vi "Coord window-Move to XY.vi"(8 "error in (no error)":errorcluster) -> (0 "error out":errorcluster)   [LabVIEW 2013]
uses:
  Globals/Coord window-Globals.vi
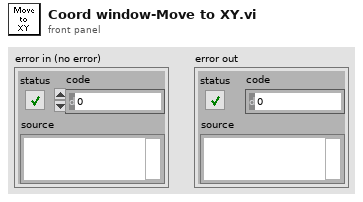
[diagram p1: front panel]
types:
  T1 = typedef "Coordinate list window refs.ctl" = cluster{"Window Name (i.e. Key)":string, "menu reference":refnum<k9>, "VI's reference":refnum<vi>, "Pane 1":refnum<vi>, "Pane 2":refnum<vi>, "Coord Listbox":refnum<vi>, "File name":refnum<vi>, "Picture Map":refnum<vi>, "Stage XYZ Position ind.":refnum<vi>}
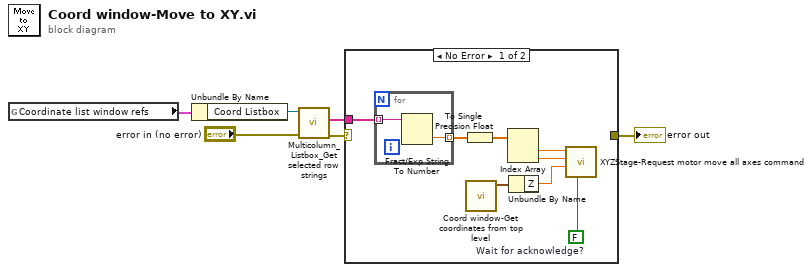
[diagram p0: block diagram]
diagram:
  n1 = global read "Coord window-Globals.vi" "Coordinate list window refs"() -> (w5:T1)
  n2 = Unbundle By Name(w5) -> ("Coord Listbox"=w4:refnum<vi>)
  n3 = call "Multicolumn_Listbox_Get selected row strings.vi"("error in (no error)"="error in (no error)", "MulticolumnListbox in"=w4) -> ("error out"=w3:errorcluster, "Selected row strings"=w6:string[])  [unwired: 7 in, 1 out]
  n4 = case shown="No Error" w3 {
    selector: w3 -> [_ w17]
    tunnel: w6 -> [w8 _]
    tunnel: [_ w17] -> w2
    frame No Error {
      w14 = FALSE  # Wait for acknowledge?
      n5 = for {
        tunnel: w8 -> [w16] mode=indexing
        tunnel: [w15] -> w9 mode=indexing
        n6 = Fract/Exp String To Number(string=w16) -> (number=w15:dbl)  [unwired: 3 in, 1 out]
      }
      n7 = To Single Precision Float(number=w9) -> (single precision float=w11:sgl[])
      n8 = call "Coord window-Get coordinates from top level.vi"() -> ("Coordinates"=w7:cluster{"X":sgl, "Y":sgl, "Z":sgl})  [unwired: 11 in]
      n9 = Index Array(array=w11) -> (element #1=w10:sgl, element #2=w12:sgl)  [unwired: 2 in]
      n10 = Unbundle By Name(w7) -> ("Z"=w13:sgl)
      n11 = call "XYZStage-Request motor move all axes command.vi"("Wait for acknowledge?"=w14, "Motor Z"=w13, "Motor Y"=w12, "Motor X"=w10) -> ()  [unwired: 6 in, 2 out]
    }
    frame Error {
    }
  }
  "error out" <- w2
